vi "Actor Core.vi"(8 "error in":errorcluster, 11 "output_actor in":refnum<class "Output Actor.lvclass">) -> (0 "error out":errorcluster, 3 "Actor out":refnum<class "Actor.lvclass">)   [LabVIEW 2015, in "Output Actor.lvclass"]
doc: "(<B>Filename</B>: Actor Framework.lvlib:Actor.lvclass:Actor Core.vi)\n\nReceives messages to the actor, reacts to them, and initiates any error handling that may shut the actor down.\n\nDescendant classes may override this VI to append parallel tasks for the actor to complete while it handles messages. Overrides use the Call Parent Method node."
uses:
  Output Actor.lvclass
  <vilib>/ActorFramework/Actor/Actor.lvclass
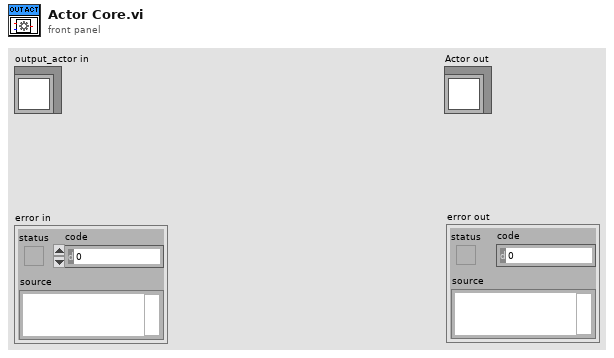
[diagram p1: front panel]
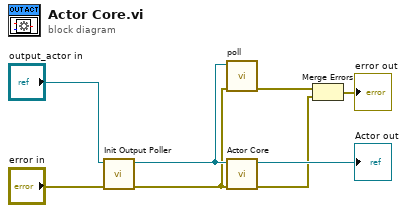
[diagram p0: block diagram]
diagram:
  n1 = call "Init Output Poller.vi"("error in (no error)"="error in", "output_actor in"="output_actor in") -> ("error out"=w1:errorcluster, "output_actor out"=w3:refnum<class "Output Actor.lvclass">)  [unwired: 8 in]
  n2 = call "poll.vi"("error in (no error)"=w1, "output_actor in"=w3) -> ("error out"=w7:errorcluster)  [unwired: 9 in]
  n3 = call-parent "Actor Core.vi"("error in"=w1, "Actor in"=w3) -> ("error out"=w6:errorcluster, "Actor out"=→"Actor out":refnum<class "Actor.lvclass">)  [unwired: 8 in]
  n4 = Merge Errors(w7, w6) -> (→"error out":errorcluster)
